vi "SinWave.vi"(9 "phase":dbl format="%.2p", 10 "amplitude":dbl=1.0 format="%0.2p", 11 "frequency":dbl=10.0 format="%0.2p") -> (3 "signal out":waveform(dbl))   [LabVIEW 2019]
uses:
  <vilib>/measure/NI_MABase.lvlib
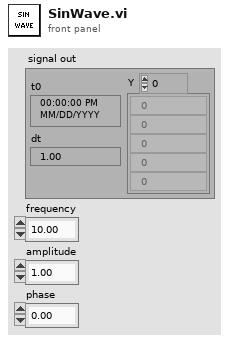
[diagram p1: front panel]
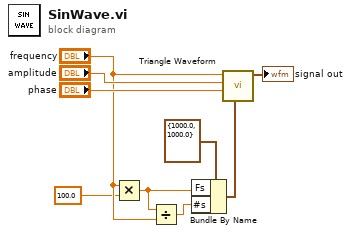
[diagram p0: block diagram]
diagram:
  n1 = Multiply(x="frequency", y=100.0) -> (x*y=w1:dbl)
  n2 = Divide(x=w1, y="frequency") -> (x/y=w3:dbl)
  n3 = Bundle By Name(cluster=cluster{"Fs":dbl, "#s":dbl} {"Fs"=1000.0, "#s"=1000.0} ("input cluster"), "Fs"=w1, "#s"=w3) -> (w2:cluster{"Fs":dbl, "#s":dbl})
  n4 = call <vilib>:"Triangle Waveform.vi"("sampling info"=w2, "phase"="phase", "amplitude"="amplitude", "frequency"="frequency") -> ("signal out"=→"signal out":waveform(dbl))  [unwired: 6 in, 1 out]
